vi "DBL Acceleration to FXP.vi"(11 "Desired acceleration (RPM/sec)":dbl min=0.0 format="%#_p") -> (0 "accel max":dbl, 1 "accel resolution":dbl, 2 "Actual acceleration (RPM/sec)":dbl min=0.0 format="%#_p", 3 "FXP acceleration":fxp<+,18,-20>, 4 "accel min":dbl)   [LabVIEW 2013, in "Engine Simulation Toolkit System Explorer.lvlib"]
uses:
  Engine Simulation Toolkit System Explorer.lvlib
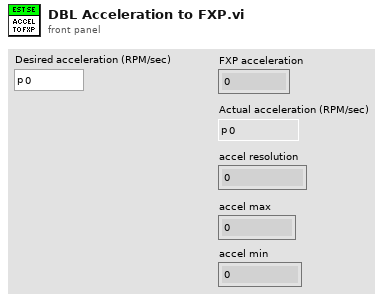
[diagram p1: front panel]
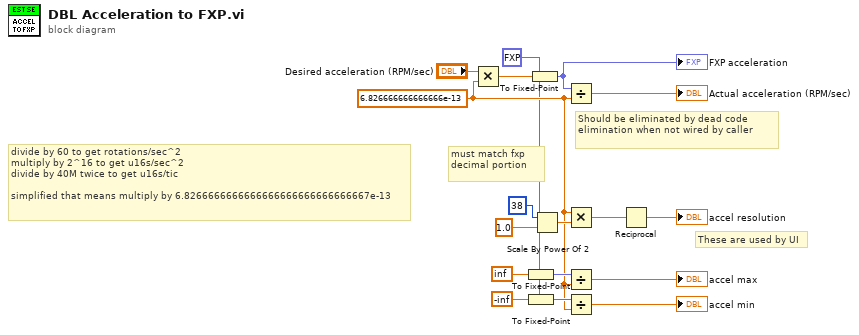
[diagram p0: block diagram]
diagram:
  w2 = 6.826666666666666e-13 ("y")
  w1 = fxp<+,18,-20> 0.0 ("u16s per tic per tic")
  # "These are used by UI"
  # "must match fxp decimal portion"
  # "Should be eliminated by dead code elimination when not wired by caller"
  # "divide by 60 to get rotations/sec^2\nmultiply by 2^16 to get u16s/sec^2\ndivide by 40M twice to get u16s/tic\n\nsimplified that means multiply by 6.8266666666666666666666666666667e-13"
  n1 = Multiply(x="Desired acceleration (RPM/sec)", y=w2) -> (x*y=w14:dbl)
  n2 = To Fixed-Point(fixed-point type=w1, number=inf) -> (fixed-point=w6:fxp<+,18,-20>)
  n3 = To Fixed-Point(fixed-point type=w1, number=-inf) -> (fixed-point=w5:fxp<+,18,-20>)
  n4 = To Fixed-Point(fixed-point type=w1, number=w14) -> (fixed-point=w16:fxp<+,18,-20>)
  "FXP acceleration" <- w16
  n5 = Scale By Power Of 2(n=i16 38, x=1.0) -> (x*2^n=w12:dbl)
  n6 = Divide(x=w16, y=w2) -> (x/y=→"Actual acceleration (RPM/sec)":dbl)
  n7 = Multiply(x=w2, y=w12) -> (x*y=w11:dbl)
  n8 = Divide(x=w6, y=w2) -> (x/y=→"accel max":dbl)
  n9 = Divide(x=w5, y=w2) -> (x/y=→"accel min":dbl)
  n10 = Reciprocal(x=w11) -> (1/x=→"accel resolution":dbl)
